vi "Update.vi"(0 "reference in":refnum<class "Display.lvclass">, 5 "error in (no error)":errorcluster) -> (14 "reference out":refnum<class "Display.lvclass">, 19 "error out":errorcluster)   [LabVIEW 2013, in "Display.lvclass"]
uses:
  Display.lvclass
  DAQ_class/DAQ.lvclass
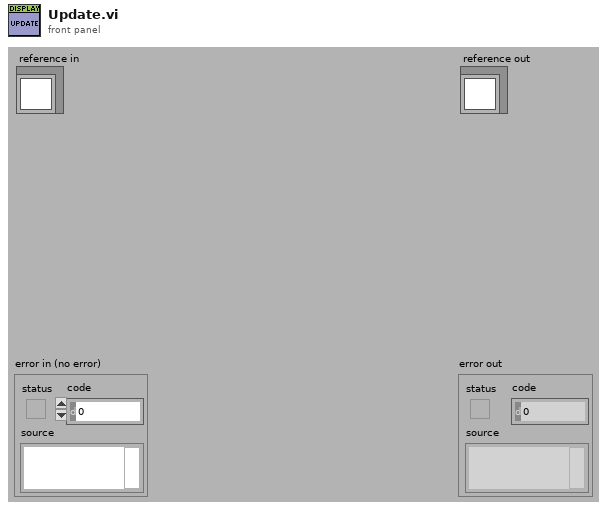
[diagram p1: front panel]
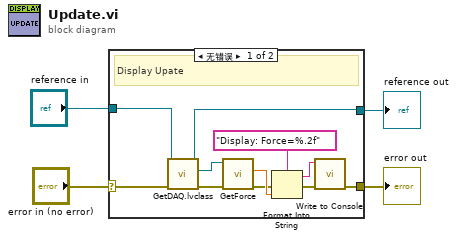
[diagram p0: block diagram]
diagram:
  n1 = case shown="无错误" "error in (no error)" {
    selector: "error in (no error)" -> [w12 w17]
    tunnel: [w8 w17] -> w3
    tunnel: [w14 w16] -> w1
    tunnel: "reference in" -> [w15 w16]
    frame No Error {
      # "Display Upate"
      n2 = call-dynamic "GetDAQ.lvclass.vi"("error in (no error)"=w12, "reference in"=w15) -> ("error out"=w11:errorcluster, "DAQ.lvclass"=w13:refnum<class "DAQ.lvclass">, "reference out"=w14:refnum<class "Display.lvclass">)  [unwired: 7 in]
      n3 = call-dynamic "GetForce.vi"("error in (no error)"=w11, "reference in"=w13) -> ("error out"=w6:errorcluster, "Force"=w7:dbl)  [unwired: 7 in, 1 out]
      n4 = Format Into String(format string="Display: Force=%.2f" ("格式字符串"), error in=w6, w7) -> (resulting string=w9:string, error out=w5:errorcluster)  [unwired: 1 in]
      n5 = call "Write to Console.vi"("error in (no error)"=w5, "Input"=w9) -> ("error out"=w8:errorcluster)  [unwired: 9 in]
    }
    frame Error {
    }
  }
  "error out" <- w3
  "reference out" <- w1
